vi "GVSDataView Set Panel Active.vi"(8 "DataView Index":i32, 11 "Selected Panel Idx In":i32) -> ()   [LabVIEW 2013]
uses:
  GVSNew View Global.vi
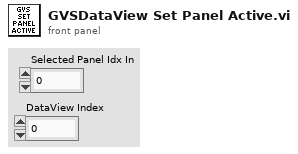
[diagram p1: front panel]
types:
  T1 = typedef "Graph Main Info Cluster.ctl" = cluster{"Selected_BarIdx":i32, "Selected_PanelIdx":i32, "Graph Main VIRef":refnum<vi>, "ToolBarClick":bool, "Spliter Ref Array":refnum<vi>[], "Panel Ref Array":refnum<vi>[], "Spliter_matrix":i32[][], "Panel_matrix":i32[][], "child_spliterIdx_matrix":i32[][], "split_pos_matrix":i32[][], "Title State":bool, "sQueueName":string, "Frame nID":i32, "Graph VIRef Array":cluster{"Graph VIRef":refnum<vi>, "Panel Idx":i32, "Frame VIRef":refnum<vi>, "Icon Ring":i32, "Graph Type":string}[], "View Type":string}
  T2 = cluster{"Graph VIRef":refnum<vi>, "Panel Idx":i32, "Frame VIRef":refnum<vi>, "Icon Ring":i32, "Graph Type":string}[]
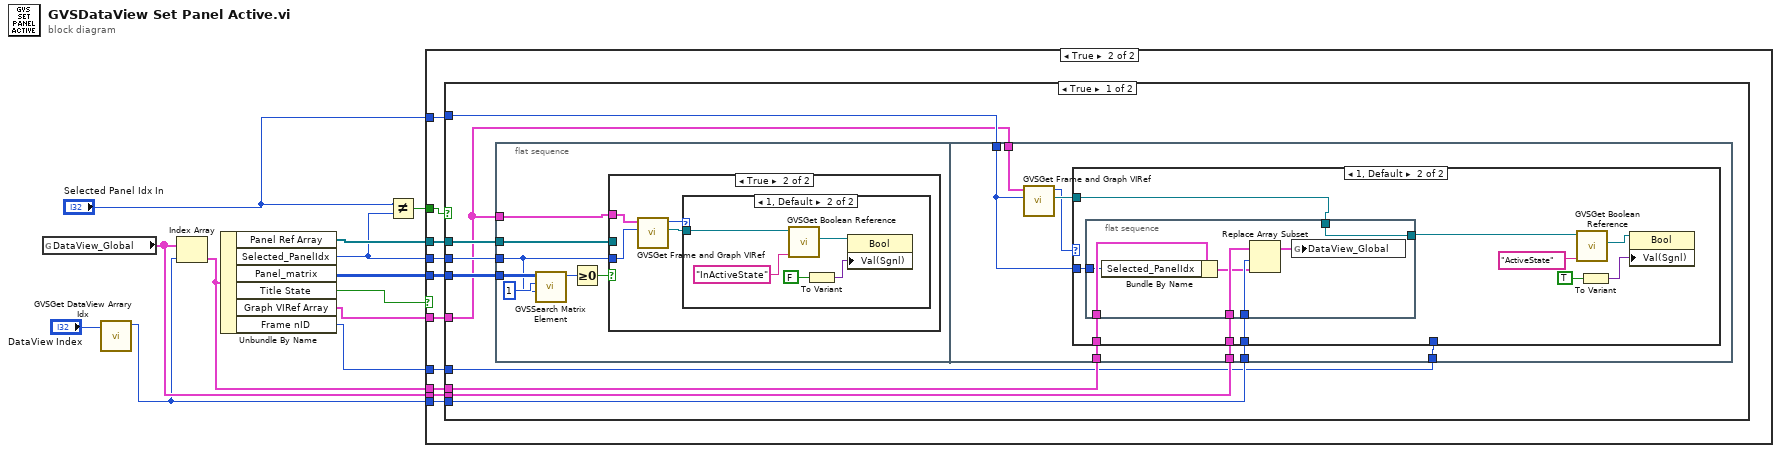
[diagram p0: block diagram]
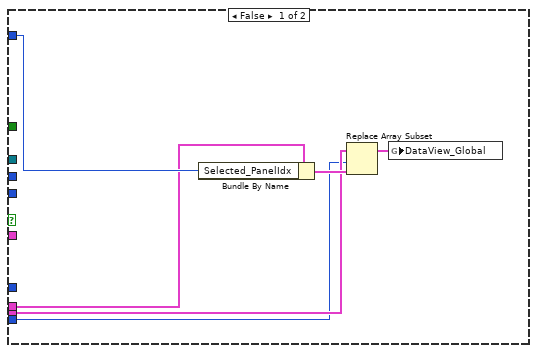
[diagram p2: hidden frame]
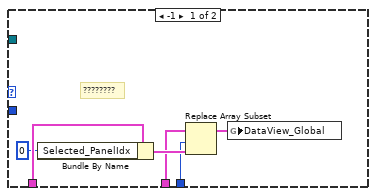
[diagram p5: hidden frame]
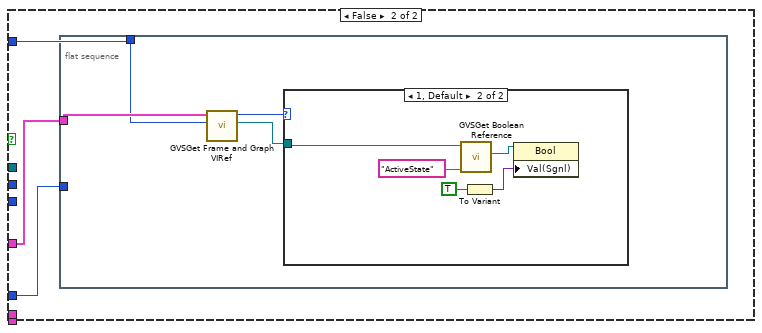
[diagram p6: hidden frame]
diagram:
  n1 = global read "GVSNew View Global.vi" "DataView_Global"() -> (w11:T1[])
  n2 = call "GVSGet DataView Arrary Idx.vi"("DataView Idx In"="DataView Index") -> ("DataView Arrary Idx out"=w7:i32)  [unwired: 10 in]
  n3 = Index Array(array=w11, index=w7) -> (element=w10:T1)
  n4 = Unbundle By Name(w10) -> ("Panel Ref Array"=w9:refnum<vi>[], "Selected_PanelIdx"=w5:i32, "Panel_matrix"=w12:i32[][], "Title State"=w3:bool, "Graph VIRef Array"=w2:T2, "Frame nID"=w1:i32)
  n5 = Not Equal?(x="Selected Panel Idx In", y=w5) -> (x != y?=w4:bool)
  n6 = case shown="True" w3 {
    tunnel: w12 -> [_ w28]
    tunnel: w11 -> [w14 w27]
    tunnel: w10 -> [w15 w26]
    tunnel: w9 -> [_ w25]
    tunnel: w7 -> [w13 w24]
    tunnel: "Selected Panel Idx In" -> [w16 w23]
    tunnel: w5 -> [_ w22]
    tunnel: w4 -> [_ w21]
    tunnel: w2 -> [_ w20]
    tunnel: w1 -> [_ w19]
    frame False {
      n7 = Bundle By Name(cluster=w15, "Selected_PanelIdx"=w16) -> (w18:T1)
      n8 = Replace Array Subset(array=w14, new element=w18, index=w13) -> (w17:T1[])
      n9 = global write "GVSNew View Global.vi" "DataView_Global"(w17) -> ()
    }
    frame True {
      n10 = case shown="True" w21 {
        tunnel: w28 -> [w37 _]
        tunnel: w27 -> [w36 _]
        tunnel: w26 -> [w35 _]
        tunnel: w25 -> [w31 _]
        tunnel: w24 -> [w34 _]
        tunnel: w23 -> [w33 w87]
        tunnel: w22 -> [w32 _]
        tunnel: w20 -> [w30 w86]
        tunnel: w19 -> [w29 w85]
        frame True {
          n11 = flat-sequence {
            tunnel: w37 -> [w44]
            tunnel: w31 -> [w40]
            tunnel: w32 -> [w39]
            tunnel: w30 -> [w38]
            tunnel: w33 -> [w57]
            tunnel: w36 -> [w61]
            tunnel: w35 -> [w60]
            tunnel: w34 -> [w59]
            tunnel: w30 -> [w58]
            tunnel: w29 -> [w54]
            frame #0 {
              n12 = call "GVSSearch Matrix Element.vi"("element"=w39, "index (row)"=1, "matrix in"=w44) -> ("index of element"=w42:i32)  [unwired: 8 in]
              n13 = Greater Or Equal To 0?(x=w42) -> (x >= 0?=w41:bool)
              n14 = case shown="True" w41 {
                tunnel: w40 -> [_ _]
                tunnel: w39 -> [_ w47]
                tunnel: w38 -> [_ w48]
                frame False {
                }
                frame True {
                  n15 = call "GVSGet Frame and Graph VIRef.vi"("Panel Idx"=w47, "Graph VIRef Array"=w48) -> ("Frame VIRef"=w46:refnum<vi>, "Graph VIRef Array Index"=w45:i32)  [unwired: 5 in, 3 out]
                  n16 = case shown="1, Default" w45 {
                    tunnel: w46 -> [_ w49]
                    frame -1 {
                    }
                    frame 1, Default {
                      n17 = call "GVSGet Boolean Reference.vi"("Label Name"="InActiveState", "VI Refnum"=w49) -> ("Boolean Ref"=w51:refnum<vi>)  [unwired: 7 in, 2 out]
                      n18 = To Variant(anything=FALSE) -> (Variant=w52:variant)
                      n19 = property class="Bool"(reference=w51, "Val(Sgnl)"=w52) -> ()  [unwired: 1 in, 2 out]
                    }
                  }
                }
              }
            }
            frame #1 {
              n20 = call "GVSGet Frame and Graph VIRef.vi"("Panel Idx"=w57, "Graph VIRef Array"=w58) -> ("Frame VIRef"=w56:refnum<vi>, "Graph VIRef Array Index"=w55:i32)  [unwired: 5 in, 3 out]
              n21 = case shown="1, Default" w55 {
                tunnel: w61 -> [w65 w77]
                tunnel: w60 -> [w63 w76]
                tunnel: w59 -> [w64 w75]
                tunnel: w57 -> [_ w74]
                tunnel: w56 -> [_ w73]
                tunnel: w54 -> [_ _]
                frame -1 {
                  # "????????"
                  n22 = Bundle By Name(cluster=w63, "Selected_PanelIdx"=0) -> (w67:T1)
                  n23 = Replace Array Subset(array=w65, new element=w67, index=w64) -> (w66:T1[])
                  n24 = global write "GVSNew View Global.vi" "DataView_Global"(w66) -> ()
                }
                frame 1, Default {
                  n25 = flat-sequence {
                    tunnel: w77 -> [w84]
                    tunnel: w76 -> [w83]
                    tunnel: w75 -> [w82]
                    tunnel: w74 -> [w81]
                    tunnel: w73 -> [w78]
                    tunnel: [w78] -> w72
                    frame #0 {
                      n26 = Bundle By Name(cluster=w83, "Selected_PanelIdx"=w81) -> (w80:T1)
                      n27 = Replace Array Subset(array=w84, new element=w80, index=w82) -> (w79:T1[])
                      n28 = global write "GVSNew View Global.vi" "DataView_Global"(w79) -> ()
                    }
                  }
                  n29 = call "GVSGet Boolean Reference.vi"("Label Name"="ActiveState", "VI Refnum"=w72) -> ("Boolean Ref"=w70:refnum<vi>)  [unwired: 7 in, 2 out]
                  n30 = To Variant(anything=TRUE) -> (Variant=w69:variant)
                  n31 = property class="Bool"(reference=w70, "Val(Sgnl)"=w69) -> ()  [unwired: 1 in, 2 out]
                }
              }
            }
          }
        }
        frame False {
          n32 = flat-sequence {
            tunnel: w87 -> [w90]
            tunnel: w86 -> [w91]
            tunnel: w85 -> [_]
            frame #0 {
              n33 = call "GVSGet Frame and Graph VIRef.vi"("Panel Idx"=w90, "Graph VIRef Array"=w91) -> ("Frame VIRef"=w89:refnum<vi>, "Graph VIRef Array Index"=w88:i32)  [unwired: 5 in, 3 out]
              n34 = case shown="1, Default" w88 {
                tunnel: w89 -> [_ w96]
                frame -1 {
                }
                frame 1, Default {
                  n35 = call "GVSGet Boolean Reference.vi"("Label Name"="ActiveState", "VI Refnum"=w96) -> ("Boolean Ref"=w94:refnum<vi>)  [unwired: 7 in, 2 out]
                  n36 = To Variant(anything=TRUE) -> (Variant=w93:variant)
                  n37 = property class="Bool"(reference=w94, "Val(Sgnl)"=w93) -> ()  [unwired: 1 in, 2 out]
                }
              }
            }
          }
        }
      }
    }
  }
